vi "Close.vi"(8 "error in (no error)":errorcluster, 11 "PostUUT in":refnum<class "PostUUT.lvclass">) -> (0 "error out":errorcluster, 3 "PostUUT out":refnum<class "PostUUT.lvclass">)   [LabVIEW 2019, in "Sequence Main.lvlib" / "PostUUT.lvclass"]
uses:
  PostUUT.lvclass
  PostUUT.lvclass/PostUUT.ctl
  Abstract UUT/Abstract UUT.lvclass
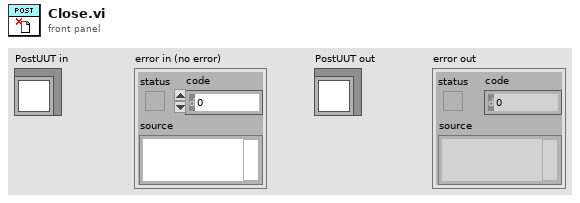
[diagram p1: front panel]
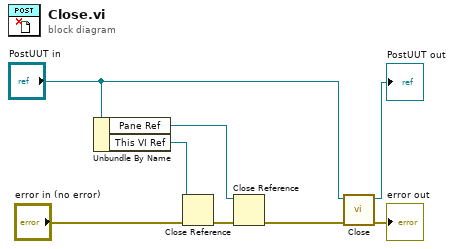
[diagram p0: block diagram]
diagram:
  n1 = Unbundle By Name("PostUUT in") -> ("Pane Ref"=w6:refnum<vi>, "This VI Ref"=w5:refnum<vi>)
  n2 = Close Reference(reference=w5, error in (no error)="error in (no error)") -> (error out=w2:errorcluster)
  n3 = Close Reference(reference=w6, error in (no error)=w2) -> (error out=w1:errorcluster)
  n4 = call-parent "Close.vi"("error in (no error)"=w1, "Abstract UUT in"="PostUUT in") -> ("error out"=→"error out":errorcluster, "Abstract UUT out"=→"PostUUT out":refnum<class "PostUUT.lvclass">)  [unwired: 8 in]
